vi "ChamberStatus (SubVI).vi"(8 "initialized array":variant[](array[variant]), 11 "JSON string":string) -> (0 "output array":variant[](array[variant]))   [LabVIEW 2017]
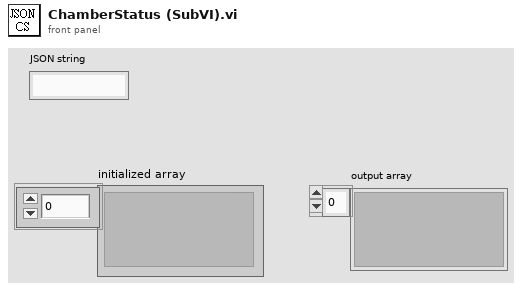
[diagram p1: front panel]
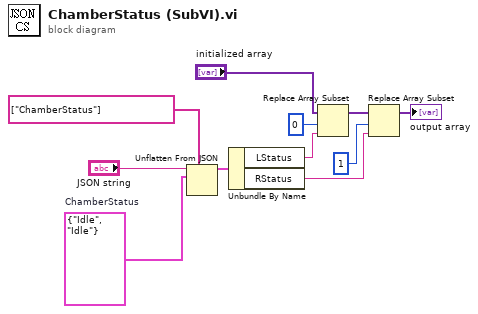
[diagram p0: block diagram]
diagram:
  w10 = cluster{"LStatus":string, "RStatus":string} {"LStatus"="Idle", "RStatus"="Idle"}  # ChamberStatus
  n1 = Unflatten From JSON(path=string[] ["ChamberStatus"], JSON string="JSON string", type and defaults=w10) -> (value=w11:cluster{"LStatus":string, "RStatus":string})  [unwired: 4 in, 1 out]
  n2 = Unbundle By Name(w11) -> ("LStatus"=w5:string, "RStatus"=w3:string)
  n3 = Replace Array Subset(array="initialized array", new element=w5, index=0) -> (w4:variant[])
  n4 = Replace Array Subset(array=w4, new element=w3, index=1) -> (→"output array":variant[])
